vi "Constants.vi"() -> ()   [LabVIEW 2019, in "RMXVisaControl Shared.lvlib"]
doc: "Use this Global VI to access the GUIDs assigned to the page resources of the Custom Device."
uses:
  RMXVisaControl Shared.lvlib
panel:
  in  "Tab Control":enum32{"GUIDS", "Constants", "Properties"}(tab)
  in  "Outputs":string="fc0c82ab-7276-4263-9317-f61f9439e937"
  in  "Inputs":string="fc0c82ab-7276-4263-9317-f61f9439e936"
  in  "RMXVisaControl":string="fc0c82ab-7276-4263-9317-f61f9439e935"
  in  "Operation Mode":string="Operation_Mode"
  in  "VISA res":string="VISA_res"
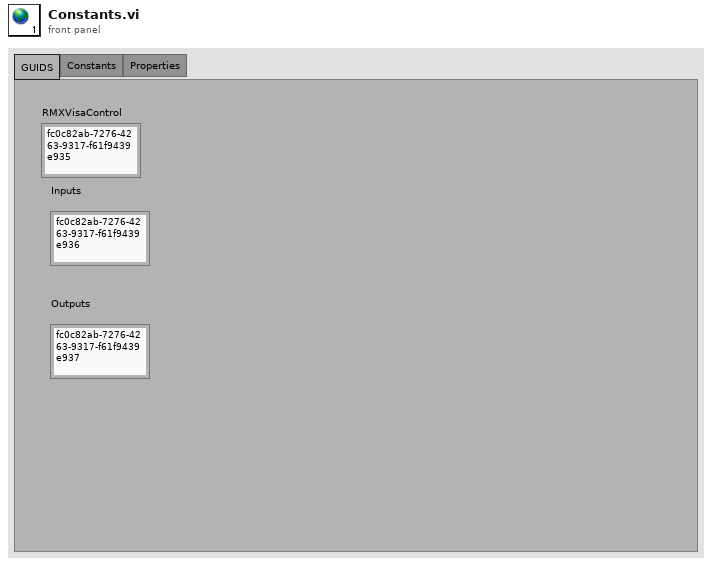
[diagram p1: front panel]
diagram:
